vi "报告存储.vi"(11 "试验时间":timestamp) -> ()   [LabVIEW 2010]
uses:
  全局量/试验配置信息.vi
  全局量/自动测试结果.vi
  全局量/全局_配置.vi
panel:
  in  "序号":i32
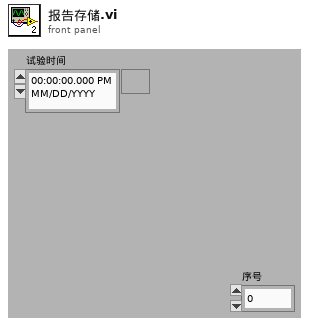
[diagram p1: front panel]
types:
  T1 = cluster{"position (Excel)":cluster{"row":i32, "column":i32}, "name (Excel)":string, "bookmark (Word)":string}
  T2 = cluster{"报告编号":string, "控制板编号":string, "控制板类型":string, "测试人员":string, "测试地点":string, string, u64, "spreadsheet string":string, "spreadsheet string":string, "spreadsheet string":string, "spreadsheet string":string}
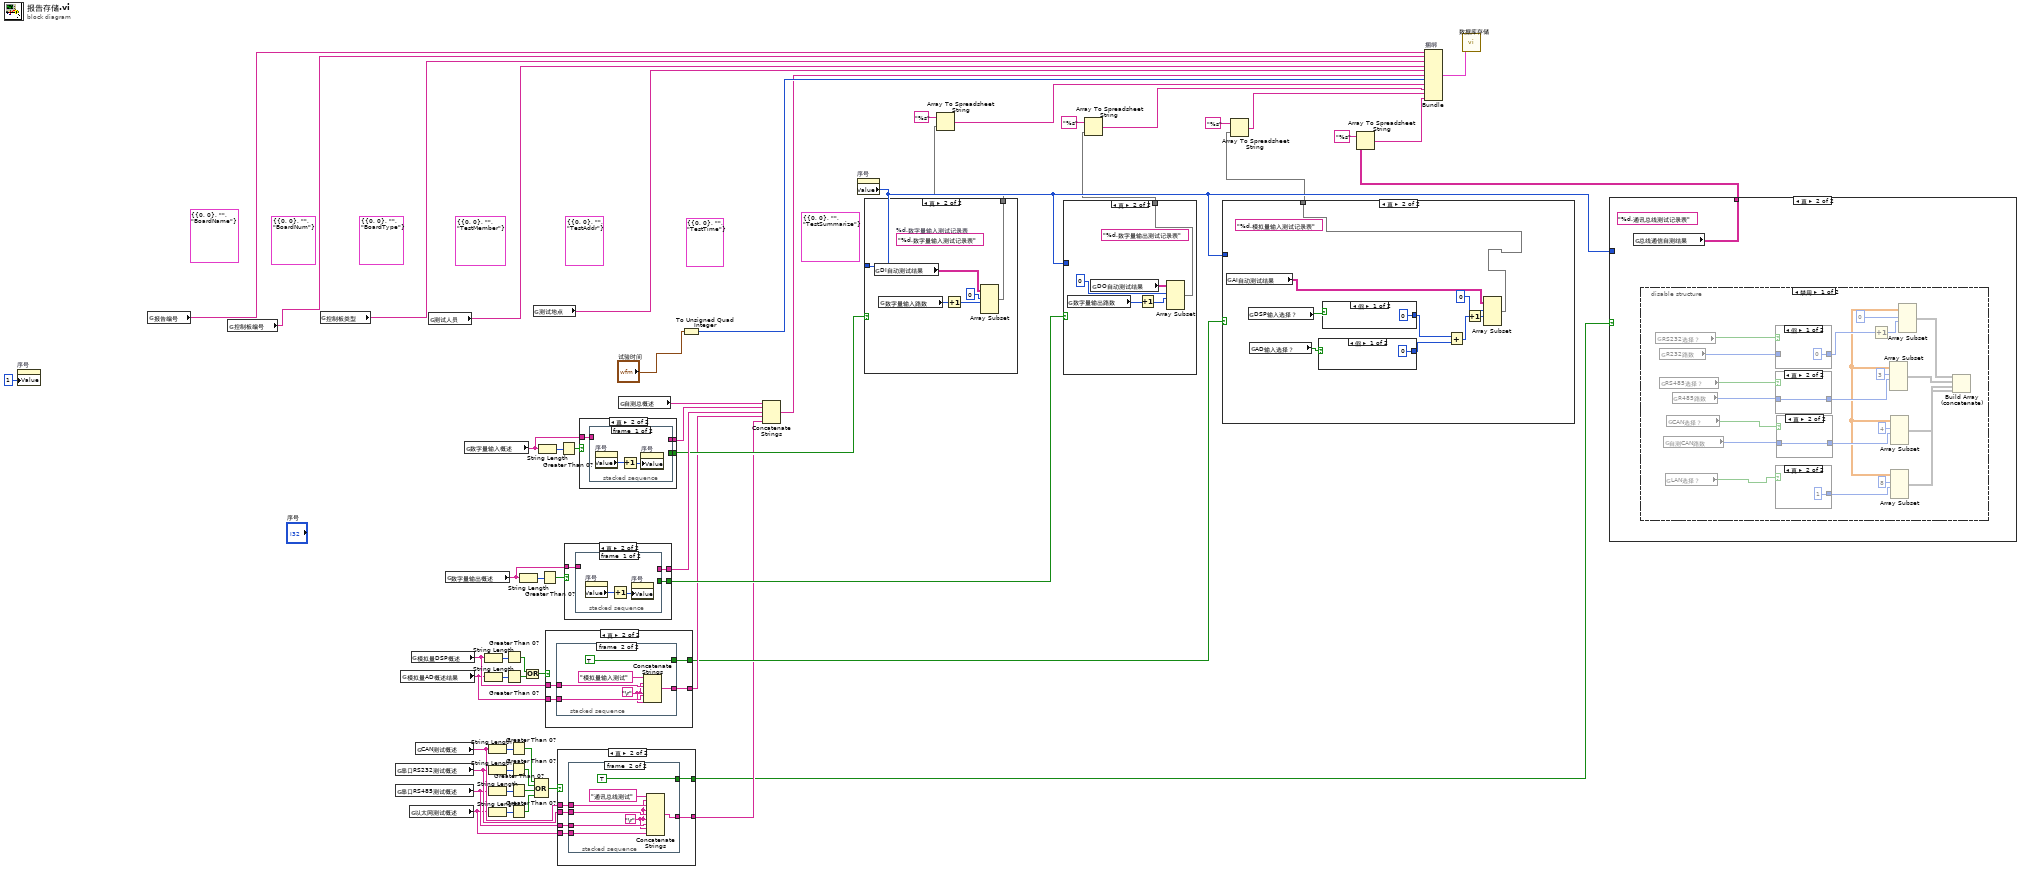
[diagram p0: block diagram]
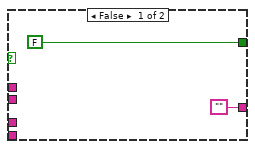
[diagram p2: hidden frame]
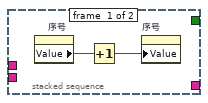
[diagram p3: hidden frame]
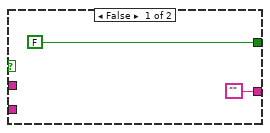
[diagram p4: hidden frame]
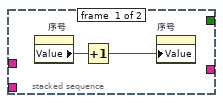
[diagram p5: hidden frame]
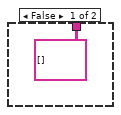
[diagram p6: hidden frame]
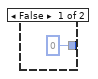
[diagram p7: hidden frame]
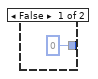
[diagram p8: hidden frame]
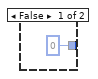
[diagram p9: hidden frame]
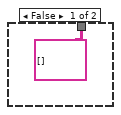
[diagram p12: hidden frame]
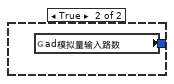
[diagram p13: hidden frame]
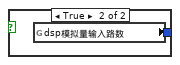
[diagram p14: hidden frame]
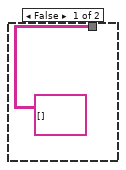
[diagram p15: hidden frame]
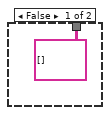
[diagram p16: hidden frame]
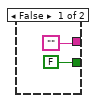
[diagram p17: hidden frame]
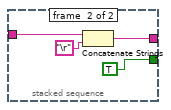
[diagram p18: hidden frame]
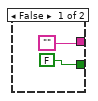
[diagram p19: hidden frame]
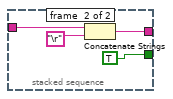
[diagram p20: hidden frame]
diagram:
  (unwired) T1 {"position (Excel)"={"row"=0, "column"=0}, "name (Excel)"="", "bookmark (Word)"="TestSummarize"} ("MS Office parameters")
  (unwired) T1 {"position (Excel)"={"row"=0, "column"=0}, "name (Excel)"="", "bookmark (Word)"="TestAddr"} ("MS Office parameters")
  (unwired) T1 {"position (Excel)"={"row"=0, "column"=0}, "name (Excel)"="", "bookmark (Word)"="TestMember"} ("MS Office parameters")
  (unwired) T1 {"position (Excel)"={"row"=0, "column"=0}, "name (Excel)"="", "bookmark (Word)"="BoardType"} ("MS Office parameters")
  (unwired) T1 {"position (Excel)"={"row"=0, "column"=0}, "name (Excel)"="", "bookmark (Word)"="BoardNum"} ("MS Office parameters")
  (unwired) T1 {"position (Excel)"={"row"=0, "column"=0}, "name (Excel)"="", "bookmark (Word)"="TestTime"} ("MS Office parameters")
  (unwired) T1 {"position (Excel)"={"row"=0, "column"=0}, "name (Excel)"="", "bookmark (Word)"="BoardName"} ("MS Office parameters")
  n1 = property on="序号" class="DigNum (严格)"("Value"=1 ("序号")) -> ()  [unwired: 2 in, 2 out]
  n2 = global read "试验配置信息.vi" "报告编号"() -> (w44:string)
  n3 = global read "试验配置信息.vi" "控制板编号"() -> (w43:string)
  n4 = global read "试验配置信息.vi" "控制板类型"() -> (w42:string)
  n5 = global read "自动测试结果.vi" "串口RS232测试概述"() -> (w6:string)
  n6 = global read "自动测试结果.vi" "串口RS485测试概述"() -> (w5:string)
  n7 = global read "自动测试结果.vi" "模拟量AD概述结果"() -> (w19:string)
  n8 = global read "自动测试结果.vi" "以太网测试概述"() -> (w4:string)
  n9 = global read "自动测试结果.vi" "模拟量DSP概述"() -> (w20:string)
  n10 = global read "自动测试结果.vi" "CAN测试概述"() -> (w7:string)
  n11 = global read "试验配置信息.vi" "测试人员"() -> (w41:string)
  n12 = global read "自动测试结果.vi" "数字量输出概述"() -> (w55:string)
  n13 = global read "自动测试结果.vi" "数字量输入概述"() -> (w56:string)
  n14 = String Length(string=w20) -> (length=w24:i32)
  n15 = String Length(string=w19) -> (length=w22:i32)
  n16 = String Length(string=w7) -> (length=w13:i32)
  n17 = String Length(string=w6) -> (length=w14:i32)
  n18 = String Length(string=w5) -> (length=w15:i32)
  n19 = String Length(string=w4) -> (length=w16:i32)
  n20 = Greater Than 0?(x=w24) -> (x > 0?=w23:bool)
  n21 = Greater Than 0?(x=w22) -> (x > 0?=w21:bool)
  n22 = Greater Than 0?(x=w13) -> (x > 0?=w12:bool)
  n23 = Greater Than 0?(x=w14) -> (x > 0?=w11:bool)
  n24 = Greater Than 0?(x=w15) -> (x > 0?=w10:bool)
  n25 = Greater Than 0?(x=w16) -> (x > 0?=w9:bool)
  n26 = String Length(string=w55) -> (length=w53:i32)
  n27 = Or(x=w23, y=w21) -> (x .or. y?=w25:bool)
  n28 = global read "试验配置信息.vi" "测试地点"() -> (w40:string)
  n29 = Compound Arithmetic op=OR(w12, w11, w10, w9) -> (w8:bool)
  n30 = String Length(string=w56) -> (length=w58:i32)
  n31 = Greater Than 0?(x=w53) -> (x > 0?=w54:bool)
  n32 = case shown="真" w25 {
    tunnel: ["" w62] -> w18
    tunnel: w20 -> [_ w64]
    tunnel: w19 -> [_ w63]
    tunnel: [FALSE w61] -> w17
    frame False {
    }
    frame True {
      n33 = stacked-sequence {
        tunnel: w64 -> [_ w72]
        tunnel: w63 -> [_ w71]
        tunnel: [_ w70] -> w62
        tunnel: [_ TRUE] -> w61
        frame #0 {
          n34 = property on="序号" class="DigNum (严格)"() -> ("Value"=w66:i32)  [unwired: 2 in, 2 out]
          n35 = Increment(x=w66) -> (x+1=w65:i32)
          n36 = property on="序号" class="DigNum (严格)"("Value"=w65) -> ()  [unwired: 2 in, 2 out]
        }
        frame #1 {
          w68 = "\r"
          n37 = Concatenate Strings("模拟量输入测试", w68, w72, w68, w71, w68) -> (w70:string)
        }
      }
    }
  }
  n38 = case shown="真" w8 {
    tunnel: ["" w76] -> w3
    tunnel: [FALSE w75] -> w2
    tunnel: w7 -> [_ w80]
    tunnel: w6 -> [_ w79]
    tunnel: w5 -> [_ w78]
    tunnel: w4 -> [_ w77]
    frame False {
    }
    frame True {
      n39 = stacked-sequence {
        tunnel: w80 -> [_ w89]
        tunnel: w79 -> [_ w88]
        tunnel: w78 -> [_ w87]
        tunnel: w77 -> [_ w86]
        tunnel: [_ w84] -> w76
        tunnel: [_ TRUE] -> w75
        frame #0 {
          n40 = property on="序号" class="DigNum (严格)"() -> ("Value"=w81:i32)  [unwired: 2 in, 2 out]
          n41 = Increment(x=w81) -> (x+1=w82:i32)
          n42 = property on="序号" class="DigNum (严格)"("Value"=w82) -> ()  [unwired: 2 in, 2 out]
        }
        frame #1 {
          w85 = "\r"
          n43 = Concatenate Strings("通讯总线测试", w85, w89, w85, w88, w85, w87, w85, w86) -> (w84:string)
        }
      }
    }
  }
  n44 = Greater Than 0?(x=w58) -> (x > 0?=w57:bool)
  n45 = case shown="真" w54 {
    tunnel: w55 -> [_ w95]
    tunnel: ["" w94] -> w50
    tunnel: [FALSE w93] -> w47
    frame False {
    }
    frame True {
      n46 = stacked-sequence {
        tunnel: w95 -> [_ w101]
        tunnel: [_ w99] -> w94
        tunnel: [_ TRUE] -> w93
        frame #0 {
          n47 = property on="序号" class="DigNum (严格)"() -> ("Value"=w97:i32)  [unwired: 2 in, 2 out]
          n48 = Increment(x=w97) -> (x+1=w96:i32)
          n49 = property on="序号" class="DigNum (严格)"("Value"=w96) -> ()  [unwired: 2 in, 2 out]
        }
        frame #1 {
          n50 = Concatenate Strings(w101, "\r") -> (w99:string)
        }
      }
    }
  }
  n51 = case shown="真" w57 {
    tunnel: w56 -> [_ w106]
    tunnel: ["" w105] -> w51
    tunnel: [FALSE w104] -> w48
    frame False {
    }
    frame True {
      n52 = stacked-sequence {
        tunnel: w106 -> [_ w112]
        tunnel: [_ w110] -> w105
        tunnel: [_ TRUE] -> w104
        frame #0 {
          n53 = property on="序号" class="DigNum (严格)"() -> ("Value"=w107:i32)  [unwired: 2 in, 2 out]
          n54 = Increment(x=w107) -> (x+1=w108:i32)
          n55 = property on="序号" class="DigNum (严格)"("Value"=w108) -> ()  [unwired: 2 in, 2 out]
        }
        frame #1 {
          n56 = Concatenate Strings(w112, "\r") -> (w110:string)
        }
      }
    }
  }
  n57 = global read "自动测试结果.vi" "自测总概述"() -> (w52:string)
  n58 = To Unsigned Quad Integer(1:"试验时间") -> (0:w39:u64)
  n59 = Concatenate Strings(w52, w51, w50, w18, w3) -> (w1:string)
  n60 = property on="序号" class="DigNum (严格)"() -> ("Value"=w46:i32)  [unwired: 2 in, 2 out]
  n61 = case shown="真" w48 {
    tunnel: w46 -> [_ _]
    tunnel: [string[][] [] ("DI自动测试结果") w117] -> w37
    frame False {
    }
    frame True {
      (unwired) "%d.数字量输入测试记录表"  # %d.数字量输入测试记录表
      n62 = global read "自动测试结果.vi" "DI自动测试结果"() -> (w116:string[][])
      n63 = global read "全局_配置.vi" "数字量输入路数"() -> (w115:i32)
      n64 = Increment(x=w115) -> (x+1=w114:i32)
      n65 = Array Subset(array=w116, index (row)=0 ("索引"), length (row)=w114) -> (w117:string[][])  [unwired: 2 in]
    }
  }
  n66 = Array To Spreadsheet String(array=w37, 3:"%s" ("格式字符串")) -> (spreadsheet string=w36:string)  [unwired: 1 in]
  n67 = case shown="真" w47 {
    tunnel: w46 -> [_ _]
    tunnel: [string[][] [] ("DO自动测试结果") w120] -> w34
    frame False {
    }
    frame True {
      (unwired) "%d.数字量输出测试记录表"
      n68 = global read "全局_配置.vi" "数字量输出路数"() -> (w124:i32)
      n69 = global read "自动测试结果.vi" "DO自动测试结果"() -> (w123:string[][])
      n70 = Increment(x=w124) -> (x+1=w122:i32)
      n71 = Array Subset(array=w123, index (row)=0 ("索引"), length (row)=w122) -> (w120:string[][])  [unwired: 2 in]
    }
  }
  n72 = Array To Spreadsheet String(array=w34, 3:"%s" ("格式字符串")) -> (spreadsheet string=w33:string)  [unwired: 1 in]
  n73 = case shown="真" w17 {
    tunnel: w46 -> [_ _]
    tunnel: [string[][] [] ("AI自动测试结果") w131] -> w31
    frame False {
    }
    frame True {
      (unwired) "%d.模拟量输入测试记录表"
      n74 = global read "自动测试结果.vi" "AI自动测试结果"() -> (w132:string[][])
      n75 = global read "试验配置信息.vi" "DSP输入选择？"() -> (w127:bool)
      n76 = global read "试验配置信息.vi" "AD输入选择？"() -> (w126:bool)
      n77 = case shown="假" w126 {
        tunnel: [u32 0 ("ad模拟量输入路数") w136] -> w130
        frame False {
        }
        frame True {
          n78 = global read "全局_配置.vi" "ad模拟量输入路数"() -> (w136:u32)
        }
      }
      n79 = case shown="假" w127 {
        tunnel: [u32 0 ("dsp模拟量输入路数") w138] -> w129
        frame False {
        }
        frame True {
          n80 = global read "全局_配置.vi" "dsp模拟量输入路数"() -> (w138:u32)
        }
      }
      n81 = Add(x=w129, y=w130) -> (x+y=w128:u32)
      n82 = Increment(x=w128) -> (x+1=w133:u32)
      n83 = Array Subset(array=w132, index (row)=0 ("索引 (行)"), length (row)=w133) -> (w131:string[][])  [unwired: 2 in]
    }
  }
  n84 = Array To Spreadsheet String(array=w31, 3:"%s" ("格式字符串")) -> (spreadsheet string=w30:string)  [unwired: 1 in]
  n85 = case shown="真" w2 {
    tunnel: w46 -> [_ _]
    tunnel: [string[][] [] ("总线通信自测结果") w140] -> w28
    frame False {
    }
    frame True {
      (unwired) "%d.通讯总线测试记录表"
      n86 = global read "自动测试结果.vi" "总线通信自测结果"() -> (w140:string[][])
      n87 = disable-structure shown="禁用" {
        frame Disabled {
          n88 = global read "试验配置信息.vi" "RS232选择？"() -> (w160:bool)
          n89 = global read "试验配置信息.vi" "RS485选择？"() -> (w158:bool)
          n90 = global read "全局_配置.vi" "R232路数"() -> (w159:u32)
          n91 = global read "试验配置信息.vi" "自测CAN路数"() -> (w155:i32)
          n92 = global read "试验配置信息.vi" "LAN选择？"() -> (w154:bool)
          n93 = global read "试验配置信息.vi" "CAN选择？"() -> (w156:bool)
          n94 = global read "全局_配置.vi" "R485路数"() -> (w157:u32)
          n95 = case shown="假" w160 {
            tunnel: w159 -> [_ w169]
            tunnel: [u32 0 ("R232路数") w169] -> w142
            frame False {
            }
            frame True {
            }
          }
          n96 = case shown="真" w158 {
            tunnel: w157 -> [_ w167]
            tunnel: [u32 0 ("R232路数") w167] -> w152
            frame False {
            }
            frame True {
            }
          }
          n97 = case shown="真" w154 {
            tunnel: [u32 0 ("R232路数") u32 1 ("R232路数")] -> w148
            frame False {
            }
            frame True {
            }
          }
          n98 = case shown="真" w156 {
            tunnel: w155 -> [_ w165]
            tunnel: [u32 0 ("R232路数") w165] -> w150
            frame False {
            }
            frame True {
            }
          }
          n99 = Increment(x=w142) -> (x+1=w143:u32)
          n100 = Array Subset(index (row)=0 ("索引"), length (row)=w143) -> (array=w141:dbl[][], w147:void[][])  [unwired: 2 in]
          n101 = Array Subset(array=w141, index (row)=3 ("索引"), length (row)=w152) -> (w146:void[][])  [unwired: 2 in]
          n102 = Array Subset(array=w141, index (row)=4 ("索引"), length (row)=w150) -> (w145:void[][])  [unwired: 2 in]
          n103 = Array Subset(array=w141, index (row)=8 ("索引"), length (row)=w148) -> (w144:void[][])  [unwired: 2 in]
          n104 = Build Array (concatenate)(w147, w146, w145, w144) -> ()  [unwired: 1 out]
        }
        frame Enabled {
        }
      }
    }
  }
  n105 = Array To Spreadsheet String(array=w28, 3:"%s" ("格式字符串")) -> (spreadsheet string=w27:string)  [unwired: 1 in]
  n106 = Bundle "捆绑"("报告编号"=w44, "控制板编号"=w43, "控制板类型"=w42, "测试人员"=w41, "测试地点"=w40, w1, w39, "spreadsheet string"=w36, "spreadsheet string"=w33, "spreadsheet string"=w30, "spreadsheet string"=w27) -> (w26:T2)  [unwired: 1 in]
  n107 = call "数据库存储.vi"("输出簇 2"=w26) -> ()  [unwired: 10 in]
